vi "Device Load.vi"(8 "error in (no error)":errorcluster, 9 "IED Name":string, 10 "CID File Name":string, 11 "SCADA in":refnum<class "SCADA.lvclass">) -> (0 "error out":errorcluster, 3 "SCADA out":refnum<class "SCADA.lvclass">)   [LabVIEW 2015, in "SCADA Core.lvlib" / "SCADA.lvclass"]
doc: "This message handles the loading of the CID file and inital communcations checks with the IED."
uses:
  SCADA.lvclass
  IED Actor/IED/IED.lvclass
  SCADA Messages/Store Measurement Msg/Store Measurement Msg.lvclass
  SCADA.lvclass/SCADA.ctl
  IED Actor/IED/IED.lvclass/IED.ctl
  Controls/Queue Selector.ctl
  <vilib>/ActorFramework/Actor/Actor.lvclass/Actor.ctl
  SCADA Abstract Messages/Device Load Status Msg/Device Load Status Msg.lvclass
  <vilib>/ActorFramework/Actor/Actor.lvclass
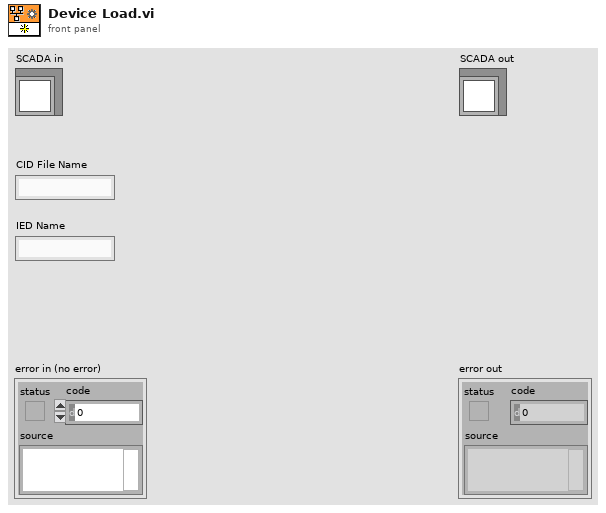
[diagram p1: front panel]
types:
  T1 = typedef "SCADA Core.lvlib/SCADA.lvclass/Queue Selector.ctl" = enum16{"IEDs", "PV", "Generators", "Wind", "Storage", "Relays"}
  T2 = typedef "NI_LVConfig.lvlib/Config Data RefNum.ctl" = refnum<k1>
  T3 = typedef "IED Actor.lvlib/IED.lvclass/Device Type Enum.ctl" = enum16{"Storage", "PV", "Generator", "Relay", "PCC", "Wind"}
  T4 = typedef "SCADA Core.lvlib/Device Load Status Msg.lvclass/Device Load Status.ctl" = enum16{"Success", "Failure"}
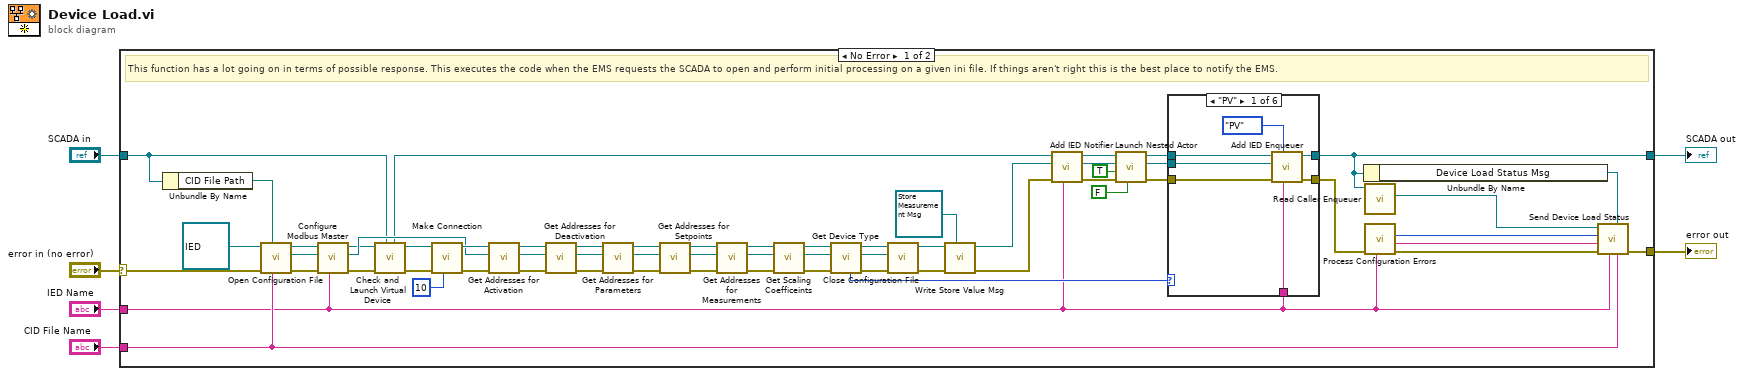
[diagram p0: block diagram]
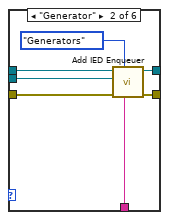
[diagram p2: hidden frame]
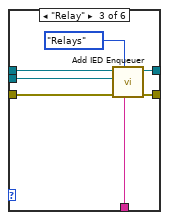
[diagram p3: hidden frame]
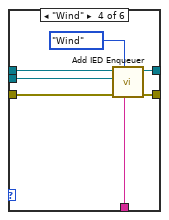
[diagram p4: hidden frame]
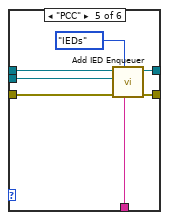
[diagram p5: hidden frame]
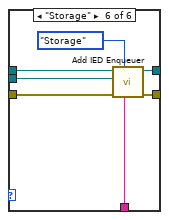
[diagram p6: hidden frame]
diagram:
  n1 = case shown="No Error" "error in (no error)" {
    selector: "error in (no error)" -> [w63 w111]
    tunnel: [w65 w111] -> w5
    tunnel: [w20 w110] -> w3
    tunnel: "SCADA in" -> [w8 w110]
    tunnel: "CID File Name" -> [w34 _]
    tunnel: "IED Name" -> [w22 _]
    frame No Error {
      # "This function has a lot going on in terms of possible response. This executes the code when the EMS requests the SCADA to open and perform initial processing on a given ini file. If things aren't right this is the best place to notify the EMS."
      n2 = Unbundle By Name(w8) -> ("CID File Path"=w35:path)
      n3 = call "Open Configuration File.vi"("Configuration File Name"=w34, "Configuration Directory Path"=w35, "error in (no error)"=w63, "IED in"=refnum<class "IED.lvclass"> refnum) -> ("error out"=w60:errorcluster, "config file refnum"=w61:T2, "IED out"=w62:refnum<class "IED.lvclass">)  [unwired: 5 in]
      n4 = call "Configure Modbus Master.vi"("IED Name"=w22, "error in (no error)"=w60, "config file refnum in"=w61, "IED in"=w62) -> ("error out"=w11:errorcluster, "config file refnum out"=w24:T2, "IED out"=w12:refnum<class "IED.lvclass">)  [unwired: 5 in]
      n5 = call "Check and Launch Virtual Device.vi"("SCADA in"=w8, "error in (no error)"=w11, "IED in"=w12) -> ("error out"=w9:errorcluster, "IED out"=w10:refnum<class "IED.lvclass">, "SCADA out"=w7:refnum<class "SCADA.lvclass">)  [unwired: 6 in]
      n6 = call "Make Connection.vi"("Number of Tries"=10, "error in (no error)"=w9, "IED in"=w10) -> ("error out"=w58:errorcluster, "IED out"=w59:refnum<class "IED.lvclass">)  [unwired: 7 in]
      n7 = call "Get Addresses for Activation.vi"("error in (no error)"=w58, "config file refnum in"=w24, "IED in"=w59) -> ("error out"=w56:errorcluster, "config file refnum out"=w55:T2, "IED out"=w57:refnum<class "IED.lvclass">)  [unwired: 6 in]
      n8 = call "Get Addresses for Deactivation.vi"("error in (no error)"=w56, "config file refnum in"=w55, "IED in"=w57) -> ("error out"=w52:errorcluster, "config file refnum out"=w53:T2, "IED out"=w54:refnum<class "IED.lvclass">)  [unwired: 6 in]
      n9 = call "Get Addresses for Parameters.vi"("error in (no error)"=w52, "config file refnum in"=w53, "IED in"=w54) -> ("error out"=w51:errorcluster, "config file refnum out"=w50:T2, "IED out"=w49:refnum<class "IED.lvclass">)  [unwired: 6 in]
      n10 = call "Get Addresses for Setpoints.vi"("error in (no error)"=w51, "config file refnum in"=w50, "IED in"=w49) -> ("error out"=w46:errorcluster, "config file refnum out"=w47:T2, "IED out"=w48:refnum<class "IED.lvclass">)  [unwired: 6 in]
      n11 = call "Get Addresses for Measurements.vi"("error in (no error)"=w46, "config file refnum in"=w47, "IED in"=w48) -> ("error out"=w43:errorcluster, "config file refnum out"=w44:T2, "IED out"=w45:refnum<class "IED.lvclass">)  [unwired: 6 in]
      n12 = call "Get Scaling Coefficeints.vi"("error in (no error)"=w43, "config file refnum in"=w44, "IED in"=w45) -> ("error out"=w42:errorcluster, "config file refnum out"=w40:T2, "IED out"=w41:refnum<class "IED.lvclass">)  [unwired: 6 in]
      n13 = call "Get Device Type.vi"("error in (no error)"=w42, "config file refnum in"=w40, "IED in"=w41) -> ("error out"=w39:errorcluster, "config file refnum out"=w37:T2, "IED out"=w38:refnum<class "IED.lvclass">, "Device Type"=w36:T3)  [unwired: 5 in]
      n14 = call "Close Configuration File.vi"("error in (no error)"=w39, "config file refnum in"=w37, "IED in"=w38) -> ("error out"=w29:errorcluster, "IED out"=w30:refnum<class "IED.lvclass">)  [unwired: 7 in]
      n15 = call "Write Store Value Msg.vi"("Store Value Msg"=refnum<class "Store Measurement Msg.lvclass"> refnum ("SCADA Core.lvlib:Store Measurement Msg.lvclass"), "error in (no error)"=w29, "IED in"=w30) -> ("error out"=w17:errorcluster, "IED out"=w16:refnum<class "IED.lvclass">)  [unwired: 7 in]
      n16 = call "Add IED Notifier.vi"("IED Name"=w22, "error in (no error)"=w17, "IED in"=w16, "SCADA in"=w7) -> ("error out"=w18:errorcluster, "IED out"=w15:refnum<class "IED.lvclass">, "SCADA out"=w21:refnum<class "SCADA.lvclass">)  [unwired: 5 in]
      n17 = call <vilib>:"Launch Nested Actor.vi"("Open Actor Core front panel? (F)"=FALSE, "error in (no error)"=w18, "Auto-stop? (T)"=TRUE, "Nested Actor"=w15, "Caller Actor in"=w21) -> ("error out"=w25:errorcluster, "Nested Actor's Enqueuer"=w26:refnum<class "Message Enqueuer.lvclass">, "Caller Actor out"=w27:refnum<class "SCADA.lvclass">)  [unwired: 4 in]
      n18 = case shown="\"PV\"" w36 {
        tunnel: w27 -> [w74 w81 w88 w95 w102 w109]
        tunnel: w25 -> [w73 w80 w87 w94 w101 w108]
        tunnel: w22 -> [w68 w75 w82 w89 w96 w103]
        tunnel: [w71 w78 w85 w92 w99 w106] -> w20
        tunnel: [w70 w77 w84 w91 w98 w105] -> w19
        tunnel: w26 -> [w69 w76 w83 w90 w97 w104]
        frame "PV" {
          n19 = call "Add IED Enqueuer.vi"("IED Name"=w68, "Queue"=Queue_Selector."PV", "error in (no error)"=w73, "IED Enqueuer"=w69, "SCADA in"=w74) -> ("error out"=w70:errorcluster, "SCADA out"=w71:refnum<class "SCADA.lvclass">)  [unwired: 5 in]
        }
        frame "Generator" {
          n20 = call "Add IED Enqueuer.vi"("IED Name"=w75, "Queue"=Queue_Selector."Generators", "error in (no error)"=w80, "IED Enqueuer"=w76, "SCADA in"=w81) -> ("error out"=w77:errorcluster, "SCADA out"=w78:refnum<class "SCADA.lvclass">)  [unwired: 5 in]
        }
        frame "Relay" {
          n21 = call "Add IED Enqueuer.vi"("IED Name"=w82, "Queue"=Queue_Selector."Relays", "error in (no error)"=w87, "IED Enqueuer"=w83, "SCADA in"=w88) -> ("error out"=w84:errorcluster, "SCADA out"=w85:refnum<class "SCADA.lvclass">)  [unwired: 5 in]
        }
        frame "Wind" {
          n22 = call "Add IED Enqueuer.vi"("IED Name"=w89, "Queue"=Queue_Selector."Wind", "error in (no error)"=w94, "IED Enqueuer"=w90, "SCADA in"=w95) -> ("error out"=w91:errorcluster, "SCADA out"=w92:refnum<class "SCADA.lvclass">)  [unwired: 5 in]
        }
        frame "PCC" {
          n23 = call "Add IED Enqueuer.vi"("IED Name"=w96, "Queue"=Queue_Selector."IEDs", "error in (no error)"=w101, "IED Enqueuer"=w97, "SCADA in"=w102) -> ("error out"=w98:errorcluster, "SCADA out"=w99:refnum<class "SCADA.lvclass">)  [unwired: 5 in]
        }
        frame "Storage" {
          n24 = call "Add IED Enqueuer.vi"("IED Name"=w103, "Queue"=Queue_Selector."Storage", "error in (no error)"=w108, "IED Enqueuer"=w104, "SCADA in"=w109) -> ("error out"=w105:errorcluster, "SCADA out"=w106:refnum<class "SCADA.lvclass">)  [unwired: 5 in]
        }
      }
      n25 = Unbundle By Name(w20) -> ("Device Load Status Msg"=w66:refnum<class "Device Load Status Msg.lvclass">)
      n26 = call <vilib>:"Read Caller Enqueuer.vi"("Actor"=w20) -> ("Caller Enqueuer"=w67:refnum<class "Message Enqueuer.lvclass">)  [unwired: 10 in]
      n27 = call "Process Configuration Errors.vi"("IED Name"=w22, "error in (no error)"=w19) -> ("error out"=w31:errorcluster, "Error String"=w32:string, "Status"=w33:T4)  [unwired: 7 in]
      n28 = call "Send Device Load Status.vi"("CID Filename"=w34, "Start Device Status Msg"=w66, "IED Name"=w22, "error in (no error)"=w31, "Error String"=w32, "Status"=w33, "Message Enqueuer in"=w67) -> ("error out"=w65:errorcluster)  [unwired: 3 in, 1 out]
    }
    frame Error {
    }
  }
  "error out" <- w5
  "SCADA out" <- w3
